vi "check hardware configuration.vi"() -> (0 "samples per pixel":i16, 1 "FPGA sample clock rate":dbl, 2 "number of lines":i32, 3 "bitfile name":T1, 4 "lasersync enable":bool)   [LabVIEW 2012]
doc: "SciScan 1.2 160622"
uses:
  Custom Controls/biotfile select.ctl
  Custom Controls/pixel resolution resonant enum.ctl
  GFG/GFGstringGet.vi
  GFG/GFGfpRefGet.vi
  GFG/GFGbooleanGet.vi
  GFG/GFGnumericGet.vi
  GFG/GFG library.lvlib
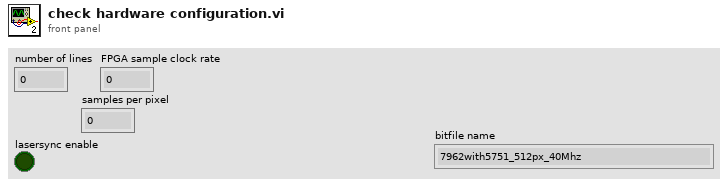
[diagram p1: front panel]
types:
  T1 = typedef "biotfile select.ctl" = enum16{"7962with5751_512px_40Mhz", "7962with5751_512px_50Mhz", "7961with5734_1024px_120Mhz or ext lasersync", "7962with5734_1024px_120Mhz or ext lasersync", "7962with5734_512px_120Mhz or ext lasersync", "7961with5734_512px_120Mhz or ext lasersync", "7962with5751_12kHz_512px_50MHz_4ch", "7962with5751_1536px_2ch_40Mhz", "7962with5751_1536px_2ch_50Mhz", "7962with5751_12kHz_1024px_2ch_50MHz"}
  T2 = typedef "pixel resolution resonant enum.ctl" = enum16{"512 x  64", "512 x 128", "512 x 256", "512 x 512", "512 x arbitrary", "1024 x 512", "1024 x 1024", " 1024 x arbitrary", " 1536 x  512", " 1536 x arbitrary"}
  T3 = cluster{"WaveformChartRef":refnum<vi>, "DigitalRef":refnum<vi>, "ArrayRef":refnum<vi>, "TabControlRef":refnum<vi>, "EnumRef":refnum<vi>, "RingRef":refnum<vi>, "BooleanRef":refnum<vi>, "KnobRef":refnum<vi>, "SlideRef":refnum<vi>, "PathRef":refnum<vi>, "StringRef":refnum<vi>, "ComboBox":refnum<vi>, "WaveformGraphRef":refnum<vi>}
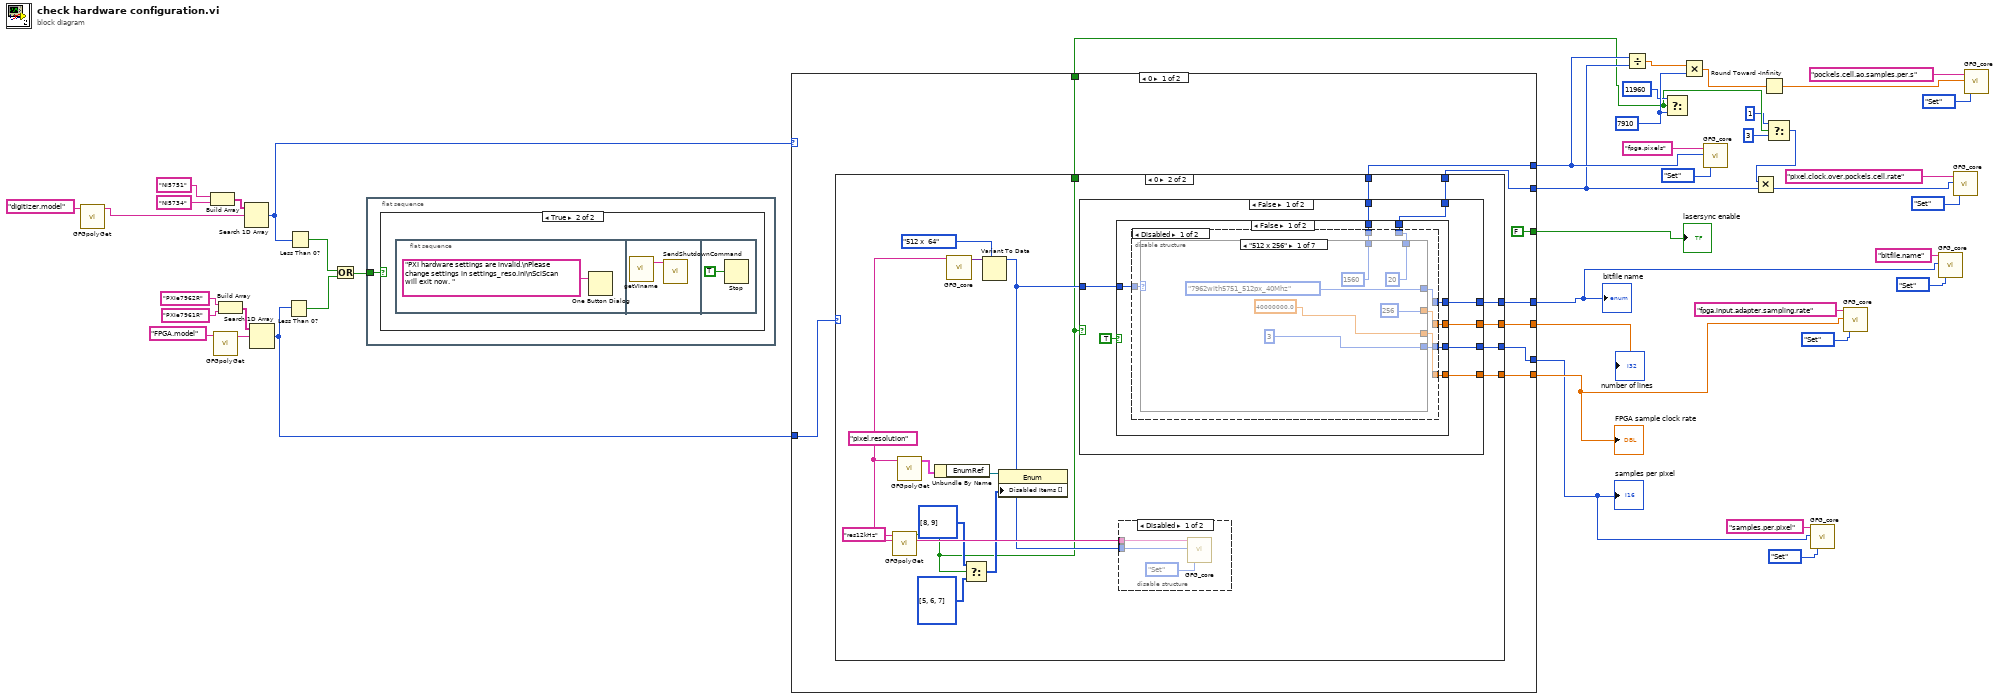
[diagram p0: block diagram]
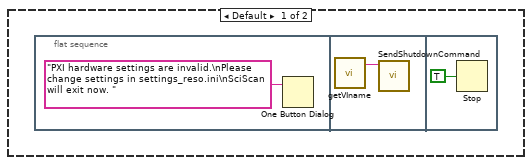
[diagram p2: hidden frame]
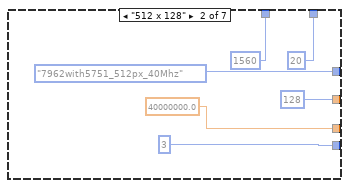
[diagram p3: hidden frame]
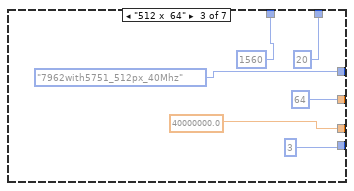
[diagram p4: hidden frame]
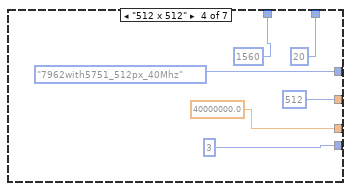
[diagram p5: hidden frame]
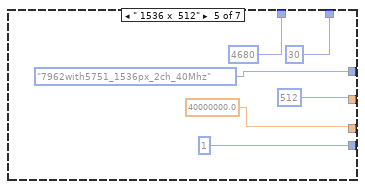
[diagram p6: hidden frame]
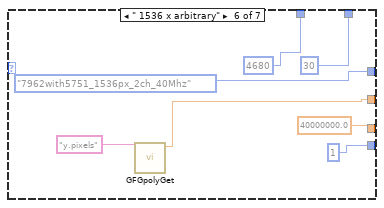
[diagram p7: hidden frame]
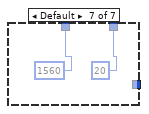
[diagram p8: hidden frame]
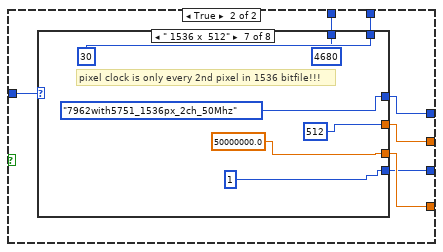
[diagram p10: hidden frame]
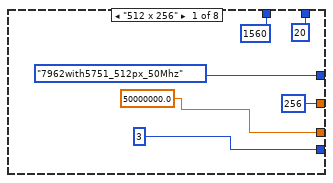
[diagram p11: hidden frame]
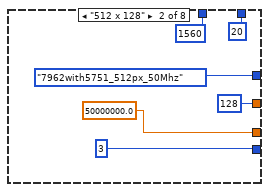
[diagram p12: hidden frame]
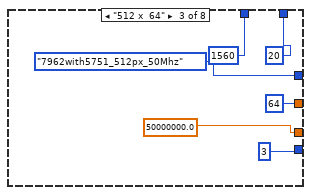
[diagram p13: hidden frame]
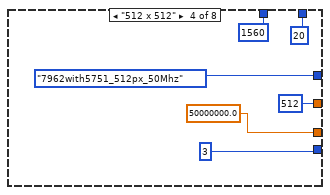
[diagram p14: hidden frame]
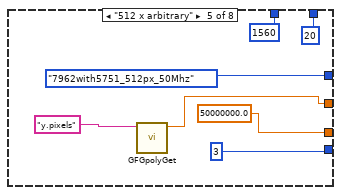
[diagram p15: hidden frame]
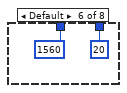
[diagram p16: hidden frame]
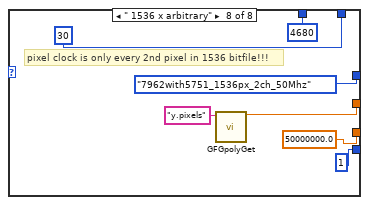
[diagram p17: hidden frame]
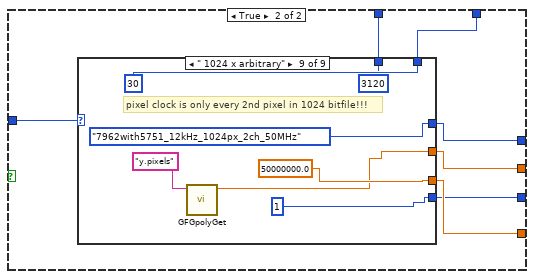
[diagram p18: hidden frame]
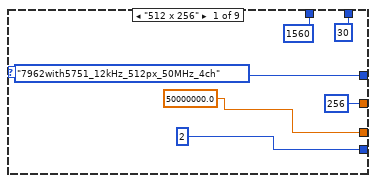
[diagram p19: hidden frame]
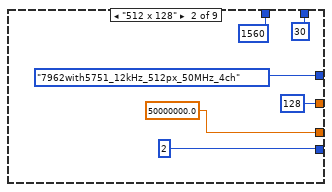
[diagram p20: hidden frame]
diagram:
  w7 = 7910
  n1 = call-poly "GFGpolyGet.vi"("Variable Name in"="digitizer.model") -> ("String"=w41:string)  [unwired: 9 in, 1 out]
  n2 = Build Array("NI5751", "NI5734") -> (w43:string[])
  n3 = call-poly "GFGpolyGet.vi"("Variable Name in"="FPGA.model") -> ("String"=w42:string)  [unwired: 9 in, 1 out]
  n4 = Build Array("PXIe7962R", "PXIe7961R") -> (w44:string[])
  n5 = Search 1D Array(1D array=w43, element=w41) -> (index of element=w31:i32)  [unwired: 1 in]
  n6 = Search 1D Array(1D array=w44, element=w42) -> (index of element=w30:i32)  [unwired: 1 in]
  n7 = Less Than 0?(x=w30) -> (x < 0?=w33:bool)
  n8 = Less Than 0?(x=w31) -> (x < 0?=w34:bool)
  n9 = Or(x=w34, y=w33) -> (x .or. y?=w32:bool)
  n10 = flat-sequence {
    tunnel: w32 -> [w45]
    frame #0 {
      n11 = case shown="True" w45 {
        frame False {
        }
        frame True {
          n12 = flat-sequence {
            frame #0 {
              n13 = One Button Dialog(message="PXI hardware settings are invalid.\nPlease change settings in settings_reso.ini\nSciScan will exit now. ") -> ()  [unwired: 1 in, 1 out]
            }
            frame #1 {
              n14 = call "getVIname.vi"() -> ("VI name"=w47:string)  [unwired: 19 in]
              n15 = call "SendShutdownCommand.vi"("Source VI"=w47) -> ()  [unwired: 11 in]
            }
            frame #2 {
              n16 = Stop(stop? (T)=TRUE) -> ()
            }
          }
        }
      }
    }
  }
  n17 = case shown="0" w31 {
    tunnel: w30 -> [w57 w265]
    tunnel: [w55 w264] -> w29
    tunnel: [w56 w263] -> w16
    tunnel: [w54 w262] -> w23
    tunnel: [w53 w261] -> w18
    tunnel: [FALSE ("Boolean") w260] -> w28
    tunnel: [w51 w259] -> w12
    tunnel: [w50 w258] -> w11
    tunnel: [w49 _] -> w4
    frame 0 {
      n18 = case shown="0" w57 {
        tunnel: [_ w75] -> w56
        tunnel: [_ w74] -> w55
        tunnel: [_ w73] -> w54
        tunnel: [_ w72] -> w53
        tunnel: [_ w68] -> w51
        tunnel: [_ w67] -> w50
        tunnel: [_ w61] -> w49
        frame Default {
          n19 = flat-sequence {
            frame #0 {
              n20 = One Button Dialog(message="PXI hardware settings are invalid.\nPlease change settings in settings_reso.ini\nSciScan will exit now. ") -> ()  [unwired: 1 in, 1 out]
            }
            frame #1 {
              n21 = call "getVIname.vi"() -> ("VI name"=w59:string)  [unwired: 19 in]
              n22 = call "SendShutdownCommand.vi"("Source VI"=w59) -> ()  [unwired: 11 in]
            }
            frame #2 {
              n23 = Stop(stop? (T)=TRUE) -> ()
            }
          }
        }
        frame 0 {
          w69 = "pixel.resolution" ("Variable Name in")
          n24 = call-poly "GFGpolyGet.vi"("Variable Name in"="res12kHz") -> ("Boolean Value OUT"=w61:bool)  [unwired: 9 in, 1 out]
          n25 = call-poly "GFGpolyGet.vi"("Variable Name in"=w69) -> ("output cluster"=w70:T3)  [unwired: 9 in, 1 out]
          n26 = Unbundle By Name(w70) -> ("EnumRef"=w71:refnum<vi>)
          n27 = call "GFG_core.vi"("Variable Name in"=w69) -> ("Variant Out"=w76:variant)  [unwired: 12 in, 6 out]
          n28 = Select(t=i32[] [8, 9] ("Disabled Items [] 2"), s=w61, f=i32[] [5, 6, 7] ("Disabled Items [] 2")) -> (s? t:f=w62:i32[])
          n29 = Variant To Data(type=pixel_resolution_resonant_enum."512 x  64" ("pixel resolution"), Variant=w76) -> (data=w66:T2)  [unwired: 1 in, 1 out]
          n30 = property class="Enum"(reference=w71, "Disabled Items []"=w62) -> ()  [unwired: 1 in, 2 out]
          n31 = case shown="False" w61 {
            tunnel: [w85 w198] -> w75
            tunnel: [w84 w197] -> w74
            tunnel: [w83 w196] -> w73
            tunnel: [w82 w195] -> w72
            tunnel: [w80 w194] -> w68
            tunnel: [w79 w193] -> w67
            tunnel: w66 -> [w78 w192]
            frame False {
              n32 = case shown="False" TRUE ("Boolean") {
                tunnel: w78 -> [w92 w145]
                tunnel: [w91 w144] -> w85
                tunnel: [w90 w143] -> w84
                tunnel: [w89 w142] -> w83
                tunnel: [w88 w141] -> w82
                tunnel: [w87 w140] -> w80
                tunnel: [w86 w139] -> w79
                frame False {
                  n33 = disable-structure shown="Disabled" {
                    disable-tunnel: w92 -> [w99 _]
                    disable-tunnel: [w98 _] -> w91
                    disable-tunnel: [w97 _] -> w90
                    disable-tunnel: [w96 _] -> w89
                    disable-tunnel: [w95 _] -> w88
                    disable-tunnel: [w94 _] -> w87
                    disable-tunnel: [w93 _] -> w86
                    frame Disabled {
                      n34 = case shown="\"512 x 256\"" w99 {
                        tunnel: [256 128 64 512 512 w132 _] -> w97
                        tunnel: [biotfile_select."7962with5751_512px_40Mhz" ("bitfile name") biotfile_select."7962with5751_512px_40Mhz" ("bitfile name") biotfile_select."7962with5751_512px_40Mhz" ("bitfile name") biotfile_select."7962with5751_512px_40Mhz" ("bitfile name") biotfile_select."7962with5751_1536px_2ch_40Mhz" ("bitfile name") biotfile_select."7962with5751_1536px_2ch_40Mhz" ("bitfile name") _] -> w98
                        tunnel: [u8 3 ("samples per pixel (internal clock)") u8 3 ("samples per pixel (internal clock)") u8 3 ("samples per pixel (internal clock)") u8 3 ("samples per pixel (internal clock)") u8 1 ("samples per pixel (internal clock)") u8 1 ("samples per pixel (internal clock)") _] -> w95
                        tunnel: [40000000.0 ("x/y") 40000000.0 ("x/y") 40000000.0 ("x/y") 40000000.0 ("x/y") 40000000.0 ("x/y") 40000000.0 ("x/y") _] -> w96
                        tunnel: [1560 1560 1560 1560 4680 4680 1560] -> w94
                        tunnel: [20 20 20 20 30 30 20] -> w93
                        frame "512 x 256" {
                        }
                        frame "512 x 128" {
                        }
                        frame "512 x  64" {
                        }
                        frame "512 x 512" {
                        }
                        frame " 1536 x  512" {
                        }
                        frame " 1536 x arbitrary" {
                          n35 = call-poly "GFGpolyGet.vi"("Variable Name in"="y.pixels") -> ("Numeric"=w132:dbl)  [unwired: 8 in, 2 out]
                        }
                        frame Default {
                        }
                      }
                    }
                    frame Enabled {
                    }
                  }
                }
                frame True {
                  n36 = case shown="\" 1536 x  512\"" w145 {
                    tunnel: [256 128 64 512 w170 _ 512 w185] -> w143
                    tunnel: [biotfile_select."7962with5751_512px_50Mhz" ("bitfile name") biotfile_select."7962with5751_512px_50Mhz" ("bitfile name") biotfile_select."7962with5751_512px_50Mhz" ("bitfile name") biotfile_select."7962with5751_512px_50Mhz" ("bitfile name") biotfile_select."7962with5751_512px_50Mhz" ("bitfile name") _ biotfile_select."7962with5751_1536px_2ch_50Mhz" ("bitfile name") biotfile_select."7962with5751_1536px_2ch_50Mhz" ("bitfile name")] -> w144
                    tunnel: [u8 3 ("samples per pixel (internal clock)") u8 3 ("samples per pixel (internal clock)") u8 3 ("samples per pixel (internal clock)") u8 3 ("samples per pixel (internal clock)") u8 3 ("samples per pixel (internal clock)") _ u8 1 ("samples per pixel (internal clock)") u8 1 ("samples per pixel (internal clock)")] -> w141
                    tunnel: [50000000.0 ("x/y") 50000000.0 ("x/y") 50000000.0 ("x/y") 50000000.0 ("x/y") 50000000.0 ("x/y") _ 50000000.0 ("x/y") 50000000.0 ("x/y")] -> w142
                    tunnel: [1560 1560 1560 1560 1560 1560 4680 4680] -> w140
                    tunnel: [20 20 20 20 20 20 30 30] -> w139
                    frame "512 x 256" {
                    }
                    frame "512 x 128" {
                    }
                    frame "512 x  64" {
                    }
                    frame "512 x 512" {
                    }
                    frame "512 x arbitrary" {
                      n37 = call-poly "GFGpolyGet.vi"("Variable Name in"="y.pixels") -> ("Numeric"=w170:dbl)  [unwired: 8 in, 2 out]
                    }
                    frame Default {
                    }
                    frame " 1536 x  512" {
                      # "pixel clock is only every 2nd pixel in 1536 bitfile!!!"
                    }
                    frame " 1536 x arbitrary" {
                      # "pixel clock is only every 2nd pixel in 1536 bitfile!!!"
                      n38 = call-poly "GFGpolyGet.vi"("Variable Name in"="y.pixels") -> ("Numeric"=w185:dbl)  [unwired: 8 in, 2 out]
                    }
                  }
                }
              }
            }
            frame True {
              n39 = case shown="\" 1024 x arbitrary\"" w192 {
                tunnel: [256 128 64 512 w223 _ 512 1024 w244] -> w197
                tunnel: [biotfile_select."7962with5751_12kHz_512px_50MHz_4ch" ("bitfile name") biotfile_select."7962with5751_12kHz_512px_50MHz_4ch" ("bitfile name") biotfile_select."7962with5751_12kHz_512px_50MHz_4ch" ("bitfile name") biotfile_select."7962with5751_12kHz_512px_50MHz_4ch" ("bitfile name") biotfile_select."7962with5751_12kHz_512px_50MHz_4ch" ("bitfile name") _ biotfile_select."7962with5751_12kHz_1024px_2ch_50MHz" ("bitfile name") biotfile_select."7962with5751_12kHz_1024px_2ch_50MHz" ("bitfile name") biotfile_select."7962with5751_12kHz_1024px_2ch_50MHz" ("bitfile name")] -> w198
                tunnel: [u8 2 ("samples per pixel (internal clock)") u8 2 ("samples per pixel (internal clock)") u8 2 ("samples per pixel (internal clock)") u8 2 ("samples per pixel (internal clock)") u8 2 ("samples per pixel (internal clock)") _ u8 1 ("samples per pixel (internal clock)") u8 1 ("samples per pixel (internal clock)") u8 1 ("samples per pixel (internal clock)")] -> w195
                tunnel: [50000000.0 ("x/y") 50000000.0 ("x/y") 50000000.0 ("x/y") 50000000.0 ("x/y") 50000000.0 ("x/y") _ 50000000.0 ("x/y") 50000000.0 ("x/y") 50000000.0 ("x/y")] -> w196
                tunnel: [1560 1560 1560 1560 1560 1560 3120 3120 3120] -> w194
                tunnel: [30 30 30 30 30 20 30 30 30] -> w193
                frame "512 x 256" {
                }
                frame "512 x 128" {
                }
                frame "512 x  64" {
                }
                frame "512 x 512" {
                }
                frame "512 x arbitrary" {
                  n40 = call-poly "GFGpolyGet.vi"("Variable Name in"="y.pixels") -> ("Numeric"=w223:dbl)  [unwired: 8 in, 2 out]
                }
                frame Default {
                }
                frame "1024 x 512" {
                  # "pixel clock is only every 2nd pixel in 1024 bitfile!!!"
                }
                frame "1024 x 1024" {
                  # "pixel clock is only every 2nd pixel in 1024 bitfile!!!"
                }
                frame " 1024 x arbitrary" {
                  # "pixel clock is only every 2nd pixel in 1024 bitfile!!!"
                  n41 = call-poly "GFGpolyGet.vi"("Variable Name in"="y.pixels") -> ("Numeric"=w244:dbl)  [unwired: 8 in, 2 out]
                }
              }
            }
          }
          n42 = disable-structure shown="Disabled" {
            disable-tunnel: w66 -> [w252 _]
            disable-tunnel: w69 -> [w251 _]
            frame Disabled {
              n43 = call "GFG_core.vi"("Variable Name in"=w251, "Variant in"=w252, "Action"=enum16{"Init", "Set", "Get", "Clear"}."Set") -> ()  [unwired: 10 in, 7 out]
            }
            frame Enabled {
            }
          }
        }
      }
    }
    frame 1, Default {
      n44 = case shown="1, Default" w265 {
        tunnel: [w272 w374] -> w264
        tunnel: [w271 w373] -> w263
        tunnel: [w270 w372] -> w262
        tunnel: [w269 w371] -> w261
        tunnel: [w268 w370] -> w260
        tunnel: [w267 w369] -> w259
        tunnel: [w266 w368] -> w258
        frame 1, Default {
          n45 = call-poly "GFGpolyGet.vi"("Variable Name in"="lasersync.enable") -> ("Boolean Value OUT"=w268:bool)  [unwired: 9 in, 1 out]
          n46 = call "GFG_core.vi"("Variable Name in"="pixel.resolution") -> ("Variant Out"=w276:variant)  [unwired: 12 in, 6 out]
          n47 = Variant To Data(type=pixel_resolution_resonant_enum."512 x  64" ("pixel resolution"), Variant=w276) -> (data=w274:T2)  [unwired: 1 in, 1 out]
          n48 = case shown="\"512 x arbitrary\"" w274 {
            tunnel: [256 128 64 512 w322 512 w345 1024] -> w272
            tunnel: [biotfile_select."7961with5734_512px_120Mhz or ext lasersync" ("bitfile name") biotfile_select."7961with5734_512px_120Mhz or ext lasersync" ("bitfile name") biotfile_select."7961with5734_512px_120Mhz or ext lasersync" ("bitfile name") biotfile_select."7961with5734_512px_120Mhz or ext lasersync" ("bitfile name") biotfile_select."7961with5734_512px_120Mhz or ext lasersync" ("bitfile name") biotfile_select."7961with5734_1024px_120Mhz or ext lasersync" ("bitfile name") biotfile_select."7961with5734_1024px_120Mhz or ext lasersync" ("bitfile name") biotfile_select."7961with5734_1024px_120Mhz or ext lasersync" ("bitfile name")] -> w271
            tunnel: w268 -> [w282 w294 w303 w314 w327 w339 w352 w362]
            tunnel: [w285 w293 w304 w316 w329 w337 w350 w360] -> w269
            tunnel: [w281 w292 w305 w315 w328 w338 w351 w361] -> w270
            tunnel: [1560 1560 1560 1560 1560 3120 3120 3120] -> w267
            tunnel: [20 20 20 20 20 40 40 40] -> w266
            frame "512 x 256" {
              n49 = Select(t=u8 5 ("samples per pixel (external clock)"), s=w282, f=u8 8 ("samples per pixel (internal clock)")) -> (s? t:f=w285:u8)
              n50 = Select(t=8000000.0 ("x/y"), s=w282, f=120000000.0 ("x/y")) -> (s? t:f=w281:dbl)
            }
            frame "512 x 128" {
              n51 = Select(t=u8 5 ("samples per pixel (external clock)"), s=w294, f=u8 8 ("samples per pixel (internal clock)")) -> (s? t:f=w293:u8)
              n52 = Select(t=8000000.0 ("x/y"), s=w294, f=120000000.0 ("x/y")) -> (s? t:f=w292:dbl)
            }
            frame "512 x  64" {
              n53 = Select(t=u8 5 ("samples per pixel (external clock)"), s=w303, f=u8 8 ("samples per pixel (internal clock)")) -> (s? t:f=w304:u8)
              n54 = Select(t=8000000.0 ("x/y"), s=w303, f=120000000.0 ("x/y")) -> (s? t:f=w305:dbl)
            }
            frame "512 x 512", Default {
              n55 = Select(t=u8 5 ("samples per pixel (external clock)"), s=w314, f=u8 8 ("samples per pixel (internal clock)")) -> (s? t:f=w316:u8)
              n56 = Select(t=8000000.0 ("x/y"), s=w314, f=120000000.0 ("x/y")) -> (s? t:f=w315:dbl)
            }
            frame "512 x arbitrary" {
              n57 = Select(t=u8 5 ("samples per pixel (external clock)"), s=w327, f=u8 8 ("samples per pixel (internal clock)")) -> (s? t:f=w329:u8)
              n58 = call-poly "GFGpolyGet.vi"("Variable Name in"="y.pixels") -> ("Numeric"=w322:dbl)  [unwired: 8 in, 2 out]
              n59 = Select(t=8000000.0 ("x/y"), s=w327, f=120000000.0 ("x/y")) -> (s? t:f=w328:dbl)
            }
            frame "1024 x 512" {
              n60 = Select(t=i16 2 ("samples per pixel (external clock)"), s=w339, f=i16 3 ("samples per pixel (internal clock)")) -> (s? t:f=w337:i16)
              n61 = Select(t=8000000.0 ("x/y"), s=w339, f=120000000.0 ("x/y")) -> (s? t:f=w338:dbl)
            }
            frame " 1024 x arbitrary" {
              n62 = Select(t=i16 2 ("samples per pixel (external clock)"), s=w352, f=i16 3 ("samples per pixel (internal clock)")) -> (s? t:f=w350:i16)
              n63 = Select(t=8000000.0 ("x/y"), s=w352, f=120000000.0 ("x/y")) -> (s? t:f=w351:dbl)
              n64 = call-poly "GFGpolyGet.vi"("Variable Name in"="y.pixels") -> ("Numeric"=w345:dbl)  [unwired: 8 in, 2 out]
            }
            frame "1024 x 1024" {
              n65 = Select(t=i16 2 ("samples per pixel (external clock)"), s=w362, f=i16 3 ("samples per pixel (internal clock)")) -> (s? t:f=w360:i16)
              n66 = Select(t=8000000.0 ("x/y"), s=w362, f=120000000.0 ("x/y")) -> (s? t:f=w361:dbl)
            }
          }
        }
        frame 0 {
          n67 = call-poly "GFGpolyGet.vi"("Variable Name in"="lasersync.enable") -> ("Boolean Value OUT"=w370:bool)  [unwired: 9 in, 1 out]
          n68 = call "GFG_core.vi"("Variable Name in"="pixel.resolution") -> ("Variant Out"=w378:variant)  [unwired: 12 in, 6 out]
          n69 = Variant To Data(type=pixel_resolution_resonant_enum."512 x  64" ("pixel resolution"), Variant=w378) -> (data=w376:T2)  [unwired: 1 in, 1 out]
          n70 = case shown="\"512 x 128\"" w376 {
            tunnel: [256 128 64 512 w424 512 1024 w458] -> w374
            tunnel: [biotfile_select."7962with5734_512px_120Mhz or ext lasersync" ("bitfile name") biotfile_select."7962with5734_512px_120Mhz or ext lasersync" ("bitfile name") biotfile_select."7962with5734_512px_120Mhz or ext lasersync" ("bitfile name") biotfile_select."7962with5734_512px_120Mhz or ext lasersync" ("bitfile name") biotfile_select."7962with5734_512px_120Mhz or ext lasersync" ("bitfile name") biotfile_select."7962with5734_1024px_120Mhz or ext lasersync" ("bitfile name") biotfile_select."7962with5734_1024px_120Mhz or ext lasersync" ("bitfile name") biotfile_select."7962with5734_1024px_120Mhz or ext lasersync" ("bitfile name")] -> w373
            tunnel: w370 -> [w384 w396 w405 w416 w429 w441 w452 w465]
            tunnel: [w387 w395 w406 w418 w431 w439 w450 w463] -> w371
            tunnel: [w383 w394 w407 w417 w430 w440 w451 w464] -> w372
            tunnel: [1560 1560 1560 1560 1560 3120 3120 3120] -> w369
            tunnel: [20 20 20 20 20 40 40 40] -> w368
            frame "512 x 256" {
              n71 = Select(t=u8 5 ("samples per pixel (external clock)"), s=w384, f=u8 8 ("samples per pixel (internal clock)")) -> (s? t:f=w387:u8)
              n72 = Select(t=8000000.0 ("x/y"), s=w384, f=120000000.0 ("x/y")) -> (s? t:f=w383:dbl)
            }
            frame "512 x 128" {
              n73 = Select(t=u8 5 ("samples per pixel (external clock)"), s=w396, f=u8 8 ("samples per pixel (internal clock)")) -> (s? t:f=w395:u8)
              n74 = Select(t=8000000.0 ("x/y"), s=w396, f=120000000.0 ("x/y")) -> (s? t:f=w394:dbl)
            }
            frame "512 x  64" {
              n75 = Select(t=u8 5 ("samples per pixel (external clock)"), s=w405, f=u8 8 ("samples per pixel (internal clock)")) -> (s? t:f=w406:u8)
              n76 = Select(t=8000000.0 ("x/y"), s=w405, f=120000000.0 ("x/y")) -> (s? t:f=w407:dbl)
            }
            frame "512 x 512", Default {
              n77 = Select(t=u8 5 ("samples per pixel (external clock)"), s=w416, f=u8 8 ("samples per pixel (internal clock)")) -> (s? t:f=w418:u8)
              n78 = Select(t=8000000.0 ("x/y"), s=w416, f=120000000.0 ("x/y")) -> (s? t:f=w417:dbl)
            }
            frame "512 x arbitrary" {
              n79 = Select(t=u8 5 ("samples per pixel (external clock)"), s=w429, f=u8 8 ("samples per pixel (internal clock)")) -> (s? t:f=w431:u8)
              n80 = call-poly "GFGpolyGet.vi"("Variable Name in"="y.pixels") -> ("Numeric"=w424:dbl)  [unwired: 8 in, 2 out]
              n81 = Select(t=8000000.0 ("x/y"), s=w429, f=120000000.0 ("x/y")) -> (s? t:f=w430:dbl)
            }
            frame "1024 x 512" {
              n82 = Select(t=i16 2 ("samples per pixel (external clock)"), s=w441, f=i16 3 ("samples per pixel (internal clock)")) -> (s? t:f=w439:i16)
              n83 = Select(t=8000000.0 ("x/y"), s=w441, f=120000000.0 ("x/y")) -> (s? t:f=w440:dbl)
            }
            frame "1024 x 1024" {
              n84 = Select(t=i16 2 ("samples per pixel (external clock)"), s=w452, f=i16 3 ("samples per pixel (internal clock)")) -> (s? t:f=w450:i16)
              n85 = Select(t=8000000.0 ("x/y"), s=w452, f=120000000.0 ("x/y")) -> (s? t:f=w451:dbl)
            }
            frame " 1024 x arbitrary" {
              n86 = Select(t=i16 2 ("samples per pixel (external clock)"), s=w465, f=i16 3 ("samples per pixel (internal clock)")) -> (s? t:f=w463:i16)
              n87 = call-poly "GFGpolyGet.vi"("Variable Name in"="y.pixels") -> ("Numeric"=w458:dbl)  [unwired: 8 in, 2 out]
              n88 = Select(t=8000000.0 ("x/y"), s=w465, f=120000000.0 ("x/y")) -> (s? t:f=w464:dbl)
            }
          }
        }
      }
      n89 = call-poly "GFGpolyGet.vi"("Variable Name in"="pixel.resolution") -> ("output cluster"=w255:T3)  [unwired: 9 in, 1 out]
      n90 = Unbundle By Name(w255) -> ("EnumRef"=w256:refnum<vi>)
      n91 = property class="Enum"(reference=w256, "Disabled Items []"=i32[] [8, 9] ("Disabled Items [] 2")) -> ()  [unwired: 1 in, 2 out]
    }
  }
  "number of lines" <- w29
  "bitfile name" <- w16
  "FPGA sample clock rate" <- w23
  "samples per pixel" <- w18
  "lasersync enable" <- w28
  n92 = Divide(x=w12, y=w11) -> (x/y=w10:dbl)
  n93 = Select(t=11960, s=w4, f=w7) -> ()  [unwired: 1 out]
  n94 = Multiply(x=w10, y=w7) -> (x*y=w9:dbl)
  n95 = call "GFG_core.vi"("Variable Name in"="fpga.pixels", "Variant in"=w12, "Action"=enum16{"Init", "Set", "Get", "Clear"}."Set") -> ()  [unwired: 10 in, 7 out]
  n96 = Round Toward -Infinity(1:w9) -> (0:w8:dbl)
  n97 = Select(t=1 ("x"), s=w4, f=3 ("x")) -> (s? t:f=w1:i32)
  n98 = Multiply(x=w1, y=w11) -> (x*y=w5:i32)
  n99 = call "GFG_core.vi"("Variable Name in"="samples.per.pixel", "Variant in"=w18, "Action"=enum16{"Init", "Set", "Get", "Clear"}."Set") -> ()  [unwired: 10 in, 7 out]
  n100 = call "GFG_core.vi"("Variable Name in"="fpga.input.adapter.sampling.rate", "Variant in"=w23, "Action"=enum16{"Init", "Set", "Get", "Clear"}."Set") -> ()  [unwired: 10 in, 7 out]
  n101 = call "GFG_core.vi"("Variable Name in"="bitfile.name", "Variant in"=w16, "Action"=enum16{"Init", "Set", "Get", "Clear"}."Set") -> ()  [unwired: 10 in, 7 out]
  n102 = call "GFG_core.vi"("Variable Name in"="pixel.clock.over.pockels.cell.rate", "Variant in"=w5, "Action"=enum16{"Init", "Set", "Get", "Clear"}."Set") -> ()  [unwired: 10 in, 7 out]
  n103 = call "GFG_core.vi"("Variable Name in"="pockels.cell.ao.samples.per.s", "Variant in"=w8, "Action"=enum16{"Init", "Set", "Get", "Clear"}."Set") -> ()  [unwired: 10 in, 7 out]
